vi "Actor Core.vi"(8 "error in":errorcluster, 11 "Panel in":refnum<class "Sample Panel.lvclass">) -> (0 "error out":errorcluster, 3 "Actor out":refnum<class "Actor.lvclass">)   [LabVIEW 2017, in "2. Basic Panel Actors.lvlib" / "Sample Panel.lvclass"]
doc: "Shows the Label and a log of all events for the panel.\n----\nCopyright: MGI 2016\nAuthor: Derek Trepanier"
uses:
  Sample Panel.lvclass
  D:/software/LabView_PanelManager/panel-actors/Source/Panel Actor/Panel Actor.lvclass
  <vilib>/ActorFramework/Actor/Actor.lvclass
  <vilib>/ActorFramework/Message Enqueuer/Message Enqueuer.lvclass/Message Enqueuer.ctl
  <vilib>/ActorFramework/Message Enqueuer/Enqueue.vi
  <vilib>/ActorFramework/Stop Msg/Stop Msg.lvclass
  C:/Program Files (x86)/National Instruments/LabVIEW 2017/vi.lib/ActorFramework/Message/Message.lvclass
  <vilib>/ActorFramework/Message Priority Queue/Priority Enqueue.vi
  panel-actors/Source/Panel Actor/Panel Actor.lvclass
panel:
  out "Label":string
  out "Top Level Panel":string
  in  "Show":bool
  in  "My Event Log":i32(listbox)
  in  "Show Dialog":bool
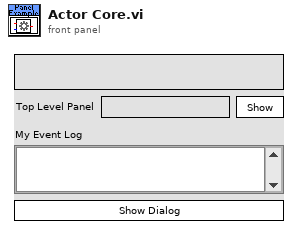
[diagram p1: front panel]
types:
  T1 = typedef "Panel.lvlib/Panel Helper.lvclass/Events.ctl" = enum16{"Initialized", "Shown", "Hidden", "Closed"}
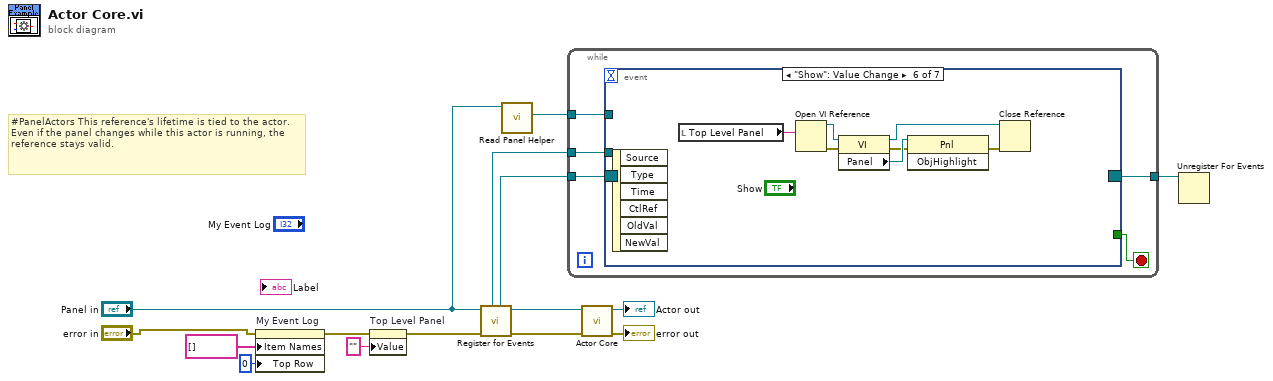
[diagram p0: block diagram]
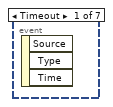
[diagram p2: hidden frame]
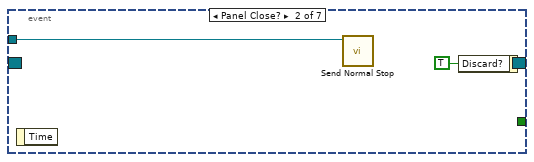
[diagram p3: hidden frame]
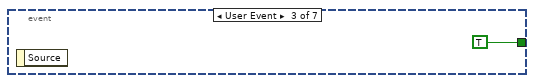
[diagram p4: hidden frame]
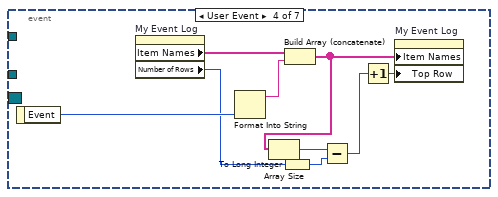
[diagram p5: hidden frame]
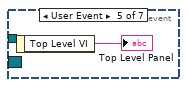
[diagram p6: hidden frame]
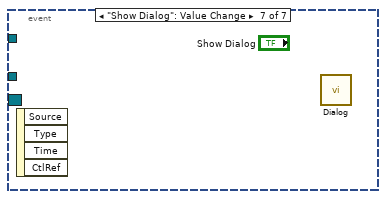
[diagram p7: hidden frame]
diagram:
  # "#PanelActors This reference's lifetime is tied to the actor. Even if the panel changes while this actor is running, the reference stays valid."
  n1 = property on="My Event Log" class="LstBox (strict)"(error in="error in", "Item Names"=string[] [], "Top Row"=0) -> (error out=w3:errorcluster)  [unwired: 1 in, 1 out]
  n2 = property on="Top Level Panel" class="Str"(error in=w3, "Value"="" ("Top Level Panel")) -> (error out=w2:errorcluster)  [unwired: 1 in, 1 out]
  n3 = call "Register for Events.vi"("Error In"=w2, "Panel Actor in"="Panel in") -> ("Error Out"=w8:errorcluster, "Panel Actor out"=w11:refnum<class "Sample Panel.lvclass">, "Pnl Actor"=w9:refnum<event-registration>, "Self Enqueuer"=w10:refnum<class "Message Enqueuer.lvclass">)  [unwired: 5 in, 1 out]
  n4 = call "Read Panel Helper.vi"("Panel Actor in"="Panel in") -> ("Panel Helper"=w7:refnum<class "Panel Helper.lvclass">)  [unwired: 9 in, 1 out]
  n5 = while {
    tunnel: w10 -> [w20]
    tunnel: w9 -> [w19]
    tunnel: w7 -> [w17]
    tunnel: [w16] -> w6
    stop <- w18 stop-if-true
    n6 = event shown="[5] \"Show\": Value Change" {
      selector: w19 -> [_ _ _ _ _ _ _]
      dyn-events: [_ _ _ _ _ _ _] -> w16
      timeout: _ -> [_ _ _ _ _ _ _]
      tunnel: w20 -> [_ w21 _ _ _ _ _]
      tunnel: [_ _ TRUE _ _ _ _] -> w18
      tunnel: w17 -> [_ _ _ _ _ _ _]
      event Timeout {
        n7 = event-data() -> ()  [unwired: 1 in, 3 out]
      }
      event Panel Close? {
        n8 = event-data() -> ()  [unwired: 1 in, 1 out]
        n9 = call <vilib>:"Send Normal Stop.vi"("Message Enqueuer"=w21) -> ()  [unwired: 10 in, 1 out]
        n10 = event-data("Discard?"=TRUE) -> ()  [unwired: 1 in, 1 out]
      }
      event User Event {
        n11 = event-data() -> ()  [unwired: 1 in, 1 out]
      }
      event User Event {
        n12 = event-data() -> ("Event"=w31:T1)  [unwired: 1 in]
        n13 = property on="My Event Log" class="LstBox (strict)"() -> ("Item Names"=w30:string[], "Number of Rows"=w28:u32)  [unwired: 2 in, 2 out]
        n14 = Format Into String(w31) -> (resulting string=w32:string)  [unwired: 3 in, 1 out]
        n15 = To Long Integer(number=w28) -> (32bit integer=w24:i32)
        n16 = Build Array (concatenate)(w30, w32) -> (w26:string[])
        n17 = Array Size(array=w26) -> (size(s)=w29:i32)
        n18 = Subtract(x=w29, y=w24) -> (x-y=w27:i32)
        n19 = Increment(x=w27) -> (x+1=w25:i32)
        n20 = property on="My Event Log" class="LstBox (strict)"("Item Names"=w26, "Top Row"=w25) -> ()  [unwired: 2 in, 2 out]
      }
      event User Event {
        n21 = event-data() -> ("Top Level VI"=→"Top Level Panel":string)  [unwired: 1 in]
      }
      event "Show": Value Change {
        n22 = event-data() -> ()  [unwired: 1 in, 6 out]
        n23 = local read "Top Level Panel"() -> (w40:string)
        n24 = Open VI Reference(vi path=w40) -> (vi reference=w39:refnum<vi>, error out=w36:errorcluster)  [unwired: 5 in]
        n25 = property class="VI"(reference=w39, error in=w36) -> (reference out=w38:refnum<vi>, error out=w35:errorcluster, "Panel"=w37:refnum<vi>)
        n26 = invoke class="Pnl" method="ObjHighlight"(reference=w37, error in=w35) -> (error out=w34:errorcluster)  [unwired: 1 in, 2 out]
        n27 = Close Reference(reference=w38, error in (no error)=w34) -> ()  [unwired: 1 out]
      }
      event "Show Dialog": Value Change {
        n28 = event-data() -> ()  [unwired: 1 in, 4 out]
        n29 = call "Dialog.vi"() -> ()  [unwired: 12 in]
      }
    }
  }
  n30 = call-parent "Actor Core.vi"("error in"=w8, "Panel Actor in"=w11) -> ("error out"=→"error out":errorcluster, "Actor out"=→"Actor out":refnum<class "Actor.lvclass">)  [unwired: 8 in]
  n31 = Unregister For Events(event registration refnum=w6) -> ()  [unwired: 1 in, 1 out]
